vi "get all aliases of a class.vi"(11 "class (eg motor)":string="motor") -> (3 "dev variable alias":string[][](array[string]))   [LabVIEW 2020]
uses:
  Preset Query Enum.ctl
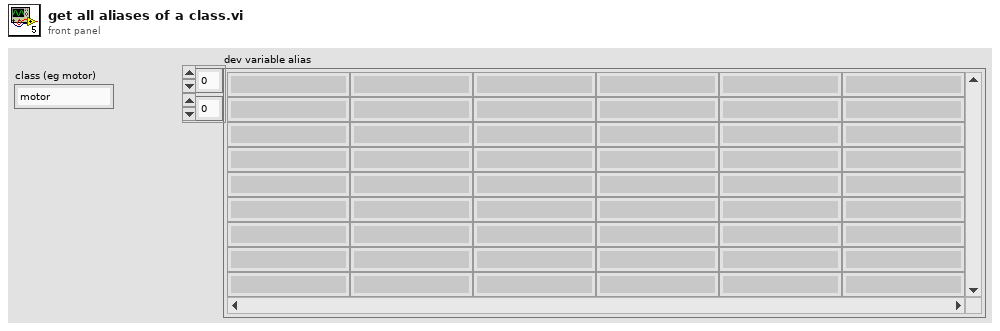
[diagram p1: front panel]
types:
  T1 = typedef "Preset Query Enum.ctl" = enum16{"Get Locations", "Get all IPs and MACs", "Get classes", "Get expt variables to set at scanstart for particular device", "Get expt devices and variables with start values", "Get expt devices and variables (with data to get)", "Get expt devices with data to get", "Get Expt devices and GUIs", "Get all devices basic properties", "Get Virtual Devices Core Info", "Get Expt names", "Get experiment basic properties", "Get experiment alarm variables", "Get MC Ports", "Get device network comm port", "Get devicetype lvclass path", "Get basic device properties", "Get Init Order", "Get all setable variables of a device", "Get device variable aliases", "Get force values of all settable variables", "Get all variables of a devicetype", "Get all variables of a device", "Get plotter details", "Get Saved Scans", "Get Scan Info", "GetGeneralGUIs", "Get expt for plotter", "Get plotter IDs from expt", "Get all devices", "Get all Virtual Devices", "Get all aliases", "Get variable and device info for Virtual Device", "GetItemLocatorIP", "Get IPs for GUIs", "Get DeviceType from Device", "GetLocalPortRange", "GetDevicePresetVariables", "Get Device Configuration", "GetAllPresetNames", "GetAllConfigurationNames", "GetPresetDeviceNames", "GetDeviceAliases", "GetDevicesOfClass"}
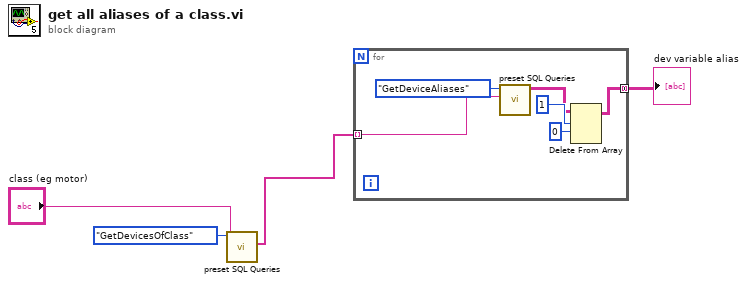
[diagram p0: block diagram]
diagram:
  n1 = call "preset SQL Queries.vi"("Device/Devicetype name\n/Plotter.id/ScanName#"="class (eg motor)", "Preset Query"=Preset_Query_Enum."GetDevicesOfClass") -> ("1st column 1st data"=w1:string[])  [unwired: 7 in, 2 out]
  n2 = for {
    tunnel: w1 -> [w9] mode=indexing
    tunnel: [w5] -> w2 mode=concatenating
    n3 = call "preset SQL Queries.vi"("Device/Devicetype name\n/Plotter.id/ScanName#"=w9, "Preset Query"=Preset_Query_Enum."GetDeviceAliases") -> ("data"=w6:string[][])  [unwired: 7 in, 2 out]
    n4 = Delete From Array(array=w6, length=1, index (row)=0 ("index")) -> (array with subset deleted=w5:string[][])  [unwired: 1 in, 1 out]
  }
  "dev variable alias" <- w2
